vi "DownloadData.vi"() -> (0 "This VI":refnum<vi>, 1 "Yaxis":dbl[](array[numeric]), 2 "Xaxis":dbl[](array[numeric]), 3 "name":string)   [LabVIEW 2020]
panel:
  in  "OK":bool
  in  "Multiplty (Iteration time)":dbl
  in  "Find Data":bool
  in  "Multiply?":bool
  out "Drata":cluster{dbl[], dbl[]}(graph)
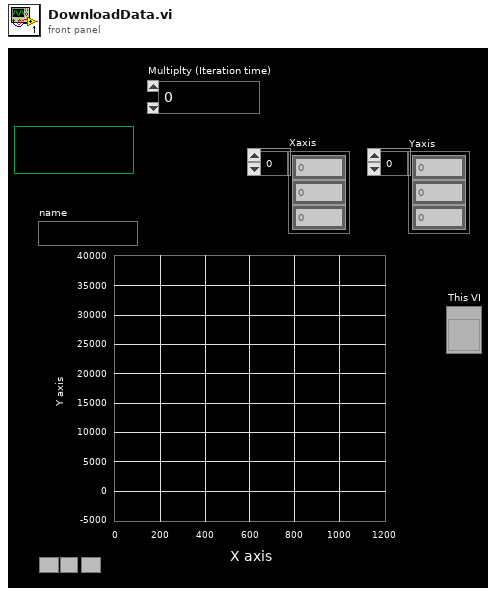
[diagram p1: front panel]
types:
  T1 = enum16{"Wait", "DownloadData", "Multiply", "Exit"}
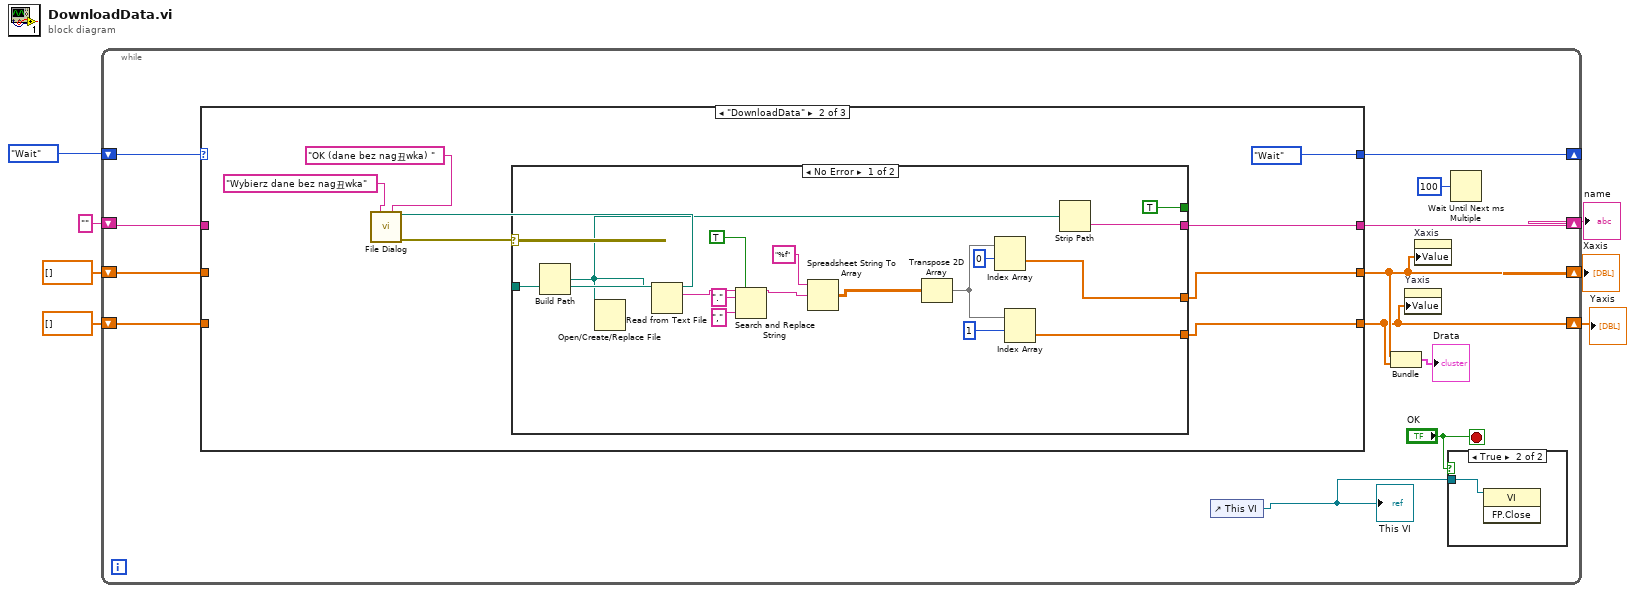
[diagram p0: block diagram]
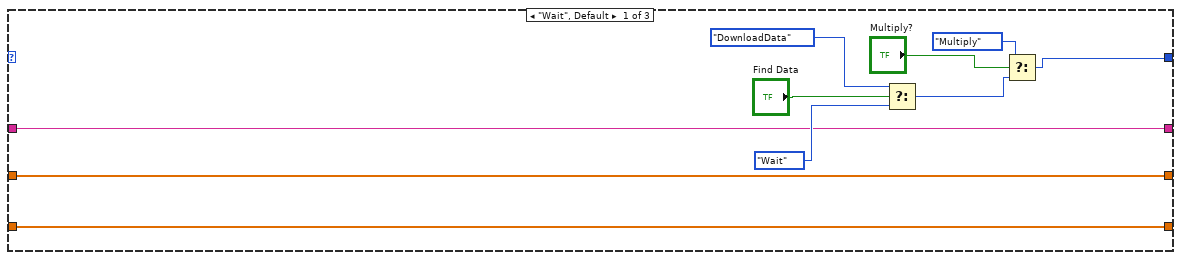
[diagram p3: hidden frame]
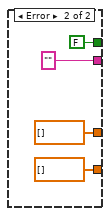
[diagram p4: hidden frame]
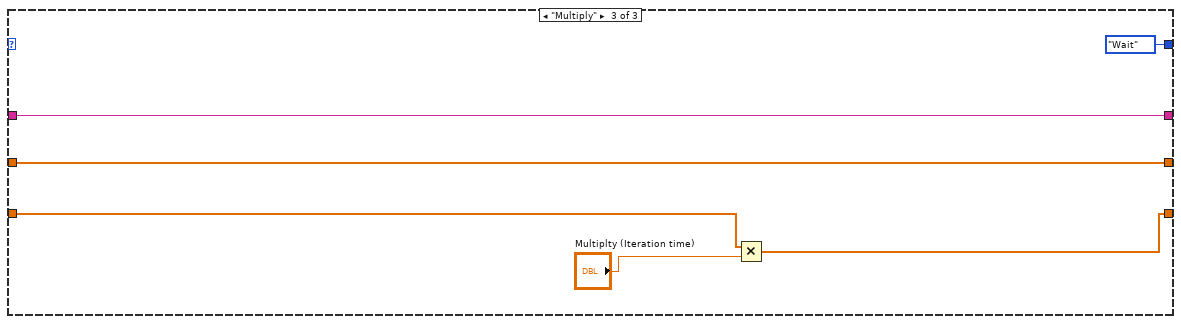
[diagram p5: hidden frame]
diagram:
  n1 = while {
    shift-right: [w12] -> w4
    shift-left: dbl[] [] -> [w14]
    shift-right: [w11] -> w6
    shift-left: dbl[] [] -> [w13]
    shift-right: [w18] -> w7
    shift-left: "" ("name") -> [w15]
    shift-right: [w17] -> _
    shift-left: T1."Wait" -> [w16]
    stop <- "OK" stop-if-true
    n2 = case shown="\"DownloadData\"" w16 {
      tunnel: [w27 w34 w64] -> w18
      tunnel: [w26 w33 w63] -> w12
      tunnel: [w25 w32 w59] -> w11
      tunnel: [w22 T1."Wait" T1."Wait"] -> w17
      tunnel: w15 -> [w27 _ w64]
      tunnel: w14 -> [w26 _ w63]
      tunnel: w13 -> [w25 _ w60]
      frame "Wait", Default {
        n3 = Select(t=T1."DownloadData", s="Find Data", f=T1."Wait") -> (s? t:f=w24:T1)
        n4 = Select(t=T1."Multiply", s="Multiply?", f=w24) -> (s? t:f=w22:T1)
      }
      frame "DownloadData" {
        n5 = call "File Dialog"("prompt"="Wybierz dane bez nag丑wka" ("button label"), "button label"="OK (dane bez nag丑wka) ") -> ("selected path"=w38:path, "error out"=w37:errorcluster)  [unwired: 10 in, 2 out]
        n6 = case shown="No Error" w37 {
          tunnel: w38 -> [w54 _]
          tunnel: [w50 "" ("name")] -> w34
          tunnel: [TRUE ("Czy dane pobrane?") FALSE ("Czy dane pobrane?")] -> _
          tunnel: [w40 dbl[] []] -> w33
          tunnel: [w39 dbl[] []] -> w32
          frame No Error {
            n7 = Build Path(name or relative path=w54) -> (appended path=w41:path)  [unwired: 1 in]
            n8 = Open/Create/Replace File(file path (use dialog)=w41) -> ()  [unwired: 5 in, 3 out]
            n9 = Read from Text File(file (use dialog)=w41) -> (text=w47:string)  [unwired: 3 in, 3 out]
            n10 = Search and Replace String(replace all?=TRUE ("replace all? (F)"), input string=w47, search string=".", replace string="," ("replace string (\"\")")) -> (result string=w43:string)  [unwired: 4 in, 3 out]
            n11 = Spreadsheet String To Array(format string="%f", spreadsheet string=w43) -> (array=w42:dbl[][])  [unwired: 2 in]
            n12 = Transpose 2D Array(2D array=w42) -> (transposed array=w51:dbl[][])
            n13 = Index Array(array=w51, index (row)=0) -> (element=w40:dbl[])  [unwired: 1 in]
            n14 = Index Array(array=w51, index (row)=1) -> (element=w39:dbl[])  [unwired: 1 in]
            n15 = Strip Path(path=w41) -> (name=w50:string)  [unwired: 1 out]
          }
          frame Error {
          }
        }
      }
      frame "Multiply" {
        n16 = Multiply(x=w60, y="Multiplty (Iteration time)") -> (x*y=w59:dbl[])
      }
    }
    n17 = control-ref of="This VI"() -> (w8:refnum<vi>)
    "This VI" <- w8
    n18 = Bundle(w12, w11) -> (→"Drata":cluster{dbl[], dbl[]})  [unwired: 1 in]
    n19 = property on="Yaxis" class="Arr (strict)"("Value"=w11) -> ()  [unwired: 2 in, 2 out]
    n20 = property on="Xaxis" class="Arr (strict)"("Value"=w12) -> ()  [unwired: 2 in, 2 out]
    n21 = case shown="True" "OK" {
      tunnel: w8 -> [_ w20]
      frame False {
      }
      frame True {
        n22 = invoke class="VI" method="FP.Close"(reference=w20) -> ()  [unwired: 2 in, 3 out]
      }
    }
    n23 = Wait Until Next ms Multiple(millisecond multiple=u32 100) -> ()  [unwired: 1 out]
  }
  "name" <- w7
  "Xaxis" <- w4
  "Yaxis" <- w6
